vi "Example 11 - In Place Element Structures.vi"   [LabVIEW 2015]
uses:
  library/Scripting.lvlib
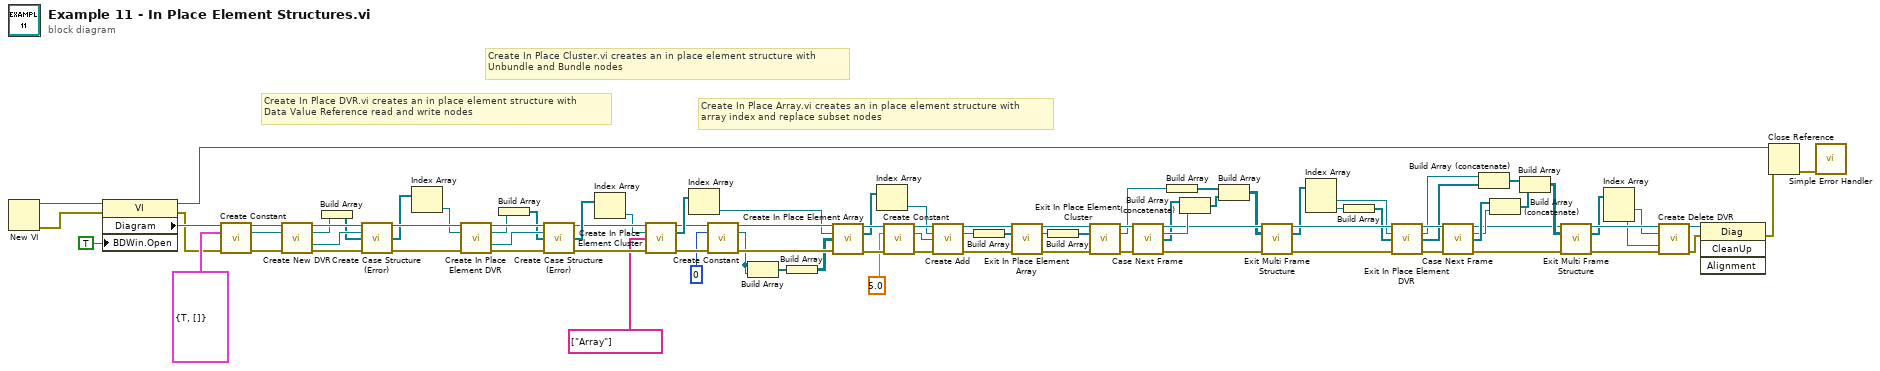
[diagram p0: block diagram]
diagram:
  # "Create In Place Array.vi creates an in place element structure with\narray index and replace subset nodes"
  # "Create In Place DVR.vi creates an in place element structure with\nData Value Reference read and write nodes"
  # "Create In Place Cluster.vi creates an in place element structure with\nUnbundle and Bundle nodes"
  n1 = New VI() -> (0:w87:errorcluster, 3:w88:refnum<vi>)  [unwired: 7 in]
  n2 = property class="VI"(reference=w88, error in=w87, "BDWin.Open"=TRUE ("Block Diagram Window:Open")) -> (reference out=w2:refnum<vi>, error out=w84:errorcluster, "Diagram"=w86:refnum<vi>)
  n3 = call "Create Constant.vi"("Diagram in"=w86, "Type"=cluster{"Boolean":bool, "Array":dbl[][]} {"Boolean"=TRUE, "Array"=[]}, "error in (no error)"=w84) -> ("Diagram out"=w83:refnum<vi>, "Terminal"=w82:refnum<vi>, "error out"=w81:errorcluster)  [unwired: 10 in]
  n4 = call "Create New DVR.vi"("Diagram in"=w83, "data value"=w82, "error in (no error)"=w81) -> ("Diagram out"=w80:refnum<vi>, "data value reference"=w77:refnum<vi>, 10:"error out"=w78:refnum<vi>, 15:"error out"=w79:errorcluster)  [unwired: 9 in]
  n5 = Build Array(w77) -> (w76:refnum<vi>[])
  n6 = call "Create Case Structure (Error).vi"("Diagram in"=w80, "Selector"=w78, "Inputs"=w76, "error in (no error)"=w79) -> ("Selected Diagram"=w75:refnum<vi>, "Inputs"=w73:refnum<vi>[], "error out"=w74:errorcluster)  [unwired: 8 in, 1 out]
  n7 = Index Array(array=w73) -> (element=w72:refnum<vi>)  [unwired: 1 in]
  n8 = call "Create In Place Element DVR.vi"("Diagram in"=w75, "DVR"=w72, "error in (no error)"=w74) -> ("Diagram out"=w71:refnum<vi>, "Data Value"=w68:refnum<vi>, "DVR Error"=w69:refnum<vi>, "error out"=w70:errorcluster)  [unwired: 8 in, 1 out]
  n9 = Build Array(w68) -> (w67:refnum<vi>[])
  n10 = call "Create Case Structure (Error).vi"("Diagram in"=w71, "Selector"=w69, "Inputs"=w67, "error in (no error)"=w70) -> ("Selected Diagram"=w65:refnum<vi>, "Inputs"=w66:refnum<vi>[], "error out"=w64:errorcluster)  [unwired: 8 in, 1 out]
  n11 = Index Array(array=w66) -> (element=w63:refnum<vi>)  [unwired: 1 in]
  n12 = call "Create In Place Element Cluster.vi"("Diagram in"=w65, "Cluster"=w63, "Element Names"=string[] ["Array"], "error in (no error)"=w64) -> ("Diagram out"=w60:refnum<vi>, "Elements"=w61:refnum<vi>[], "error out"=w59:errorcluster)  [unwired: 8 in, 1 out]
  n13 = Index Array(array=w61) -> (element=w55:refnum<vi>)  [unwired: 1 in]
  n14 = call "Create Constant.vi"("Diagram in"=w60, "Type"=0, "error in (no error)"=w59) -> ("Diagram out"=w57:refnum<vi>, "Terminal"=w54:refnum<vi>, "error out"=w56:errorcluster)  [unwired: 10 in]
  n15 = Build Array(w54, w54) -> (w53:refnum<vi>[])
  n16 = Build Array(w53) -> (w52:refnum<vi>[][])
  n17 = call "Create In Place Element Array.vi"("Diagram in"=w57, "Array"=w55, "Indices"=w52, "error in (no error)"=w56) -> ("Diagram out"=w47:refnum<vi>, "Elements"=w46:refnum<vi>[], "error out"=w51:errorcluster)  [unwired: 8 in, 1 out]
  n18 = Index Array(array=w46) -> (element=w45:refnum<vi>)  [unwired: 1 in]
  n19 = call "Create Constant.vi"("Diagram in"=w47, "Type"=5.0, "error in (no error)"=w51) -> ("Diagram out"=w49:refnum<vi>, "Terminal"=w44:refnum<vi>, "error out"=w48:errorcluster)  [unwired: 10 in]
  n20 = call "Create Add.vi"("Diagram in"=w49, "x"=w45, "y"=w44, "error in (no error)"=w48) -> ("Diagram out"=w43:refnum<vi>, "x+y"=w41:refnum<vi>, "error out"=w42:errorcluster)  [unwired: 9 in]
  n21 = Build Array(w41) -> (w40:refnum<vi>[])
  n22 = call "Exit In Place Element Array.vi"("Diagram in"=w43, "Elements"=w40, "error in (no error)"=w42) -> ("Diagram out"=w39:refnum<vi>, "Array"=w37:refnum<vi>, "error out"=w38:errorcluster)  [unwired: 8 in, 2 out]
  n23 = Build Array(w37) -> (w36:refnum<vi>[])
  n24 = call "Exit In Place Element Cluster.vi"("Diagram in"=w39, "Elements"=w36, "error in (no error)"=w38) -> ("Diagram out"=w35:refnum<vi>, "Cluster"=w33:refnum<vi>, "error out"=w34:errorcluster)  [unwired: 9 in, 1 out]
  n25 = call "Case Next Frame.vi"("Diagram in"=w35, "error in (no error)"=w34) -> ("Selected Diagram"=w29:refnum<vi>, "Selector"=w32:refnum<vi>, "Inputs"=w14:refnum<vi>[], "error out"=w27:errorcluster)  [unwired: 10 in]
  n26 = Build Array(w33) -> (w30:refnum<vi>[])
  n27 = Build Array (concatenate)(w14, w32) -> (w31:refnum<vi>[])
  n28 = Build Array(w30, w31) -> (w28:refnum<vi>[][])
  n29 = call "Exit Multi Frame Structure.vi"("Diagram in"=w29, "Outputs"=w28, "error in (no error)"=w27) -> ("Diagram out"=w26:refnum<vi>, "Outputs"=w24:refnum<vi>[], "error out"=w25:errorcluster)  [unwired: 10 in]
  n30 = Index Array(array=w24) -> (element #1=w23:refnum<vi>, element #2=w22:refnum<vi>)  [unwired: 2 in]
  n31 = Build Array(w22) -> (w21:refnum<vi>[])
  n32 = call "Exit In Place Element DVR.vi"("Diagram in"=w26, "Data Value"=w23, "Outputs"=w21, "error in (no error)"=w25) -> ("Diagram out"=w20:refnum<vi>, "DVR"=w15:refnum<vi>, "Outputs"=w1:refnum<vi>[], "error out"=w19:errorcluster)  [unwired: 7 in, 1 out]
  n33 = call "Case Next Frame.vi"("Diagram in"=w20, "error in (no error)"=w19) -> ("Selected Diagram"=w8:refnum<vi>, "Selector"=w12:refnum<vi>, "Inputs"=w13:refnum<vi>[], "error out"=w16:errorcluster)  [unwired: 10 in]
  n34 = Build Array (concatenate)(w15, w1) -> (w11:refnum<vi>[])
  n35 = Build Array (concatenate)(w13, w12) -> (w10:refnum<vi>[])
  n36 = Build Array(w11, w10) -> (w9:refnum<vi>[][])
  n37 = call "Exit Multi Frame Structure.vi"("Diagram in"=w8, "Outputs"=w9, "error in (no error)"=w16) -> ("Diagram out"=w18:refnum<vi>, "Outputs"=w7:refnum<vi>[], "error out"=w17:errorcluster)  [unwired: 10 in]
  n38 = Index Array(array=w7) -> (element #1=w6:refnum<vi>, element #2=w5:refnum<vi>)  [unwired: 2 in]
  n39 = call "Create Delete DVR.vi"("Diagram in"=w18, "data value reference"=w6, 9:"error in (no error)"=w5, 11:"error in (no error)"=w17) -> ("Diagram out"=w4:refnum<vi>, "error out"=w3:errorcluster)  [unwired: 8 in, 2 out]
  n40 = invoke class="Diag" method="CleanUp"(reference=w4, error in=w3) -> (error out=w89:errorcluster)  [unwired: 2 in, 3 out]
  n41 = Close Reference(reference=w2, error in (no error)=w89) -> (error out=w90:errorcluster)
  n42 = call <vilib>:"Simple Error Handler.vi"("error in (no error)"=w90) -> ()  [unwired: 4 in, 5 out]
